vi "E1.vi"() -> ()   [LabVIEW 2018]
panel:
  out "Waveform Chart":dynamicdata(graph)
  in  "stop (F)":bool
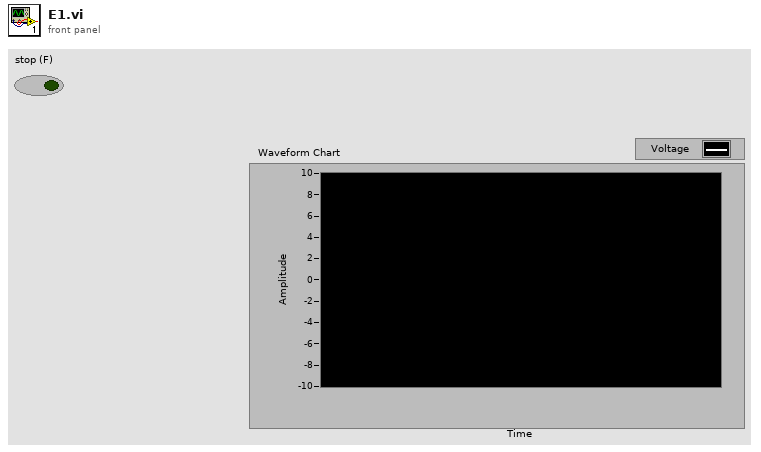
[diagram p1: front panel]
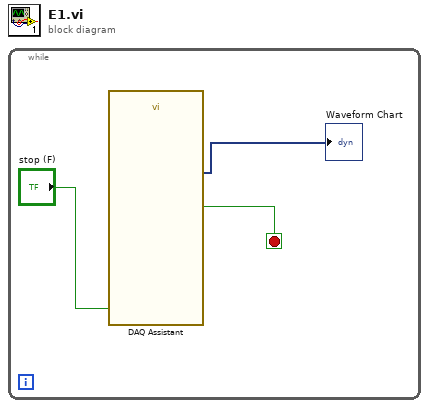
[diagram p0: block diagram]
diagram:
  n1 = while {
    stop <- w2 stop-if-true
    n2 = call "DAQ Assistant"("stop (F)"="stop (F)") -> ("data"=→"Waveform Chart":dynamicdata, "stopped"=w2:bool)  [unwired: 15 in, 2 out]
  }
